vi "字符键盘.vi"(11 "Old String":string) -> (3 "String":string)   [LabVIEW 2016, in "Alarm interface.lvlib" / "短信语音库.lvlib"]
uses:
  <vilib>/Utility/miscctls.llb/LVPointTypeDef.ctl
panel:
  in  "^":bool
  in  "$":bool
  in  "!":bool
  in  "~":bool
  in  "%":bool
  in  "&":bool
  in  "@":bool
  in  "_":bool
  in  "#":bool
  in  "大小写":bool
  in  "Z":bool
  in  "Y":bool
  in  "X":bool
  in  "W":bool
  in  "V":bool
  in  "U":bool
  in  "T":bool
  in  "S":bool
  in  "R":bool
  in  "Q":bool
  in  "P":bool
  in  "O":bool
  in  "N":bool
  in  "M":bool
  in  "L":bool
  in  "K":bool
  in  "J":bool
  in  "I":bool
  in  "H":bool
  in  "G":bool
  in  "F":bool
  in  "E":bool
  in  "D":bool
  in  "C":bool
  in  "B":bool
  in  "A":bool
  in  ",":bool
  in  "Cancel":bool
  in  "OK":bool
  in  "Clear":bool
  in  "BackSpace":bool
  in  "Point":bool
  in  "Zero":bool
  in  "Nine":bool
  in  "Eight":bool
  in  "Seven":bool
  in  "Six":bool
  in  "Five":bool
  in  "Four":bool
  in  "Three":bool
  in  "Two":bool
  in  "One":bool
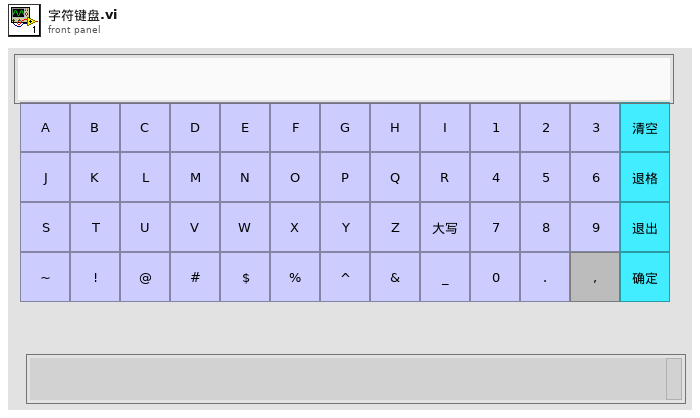
[diagram p1: front panel]
types:
  T1 = typedef "LVPointTypeDef.ctl" = cluster{"Horizontal":i16, "Vertical":i16}
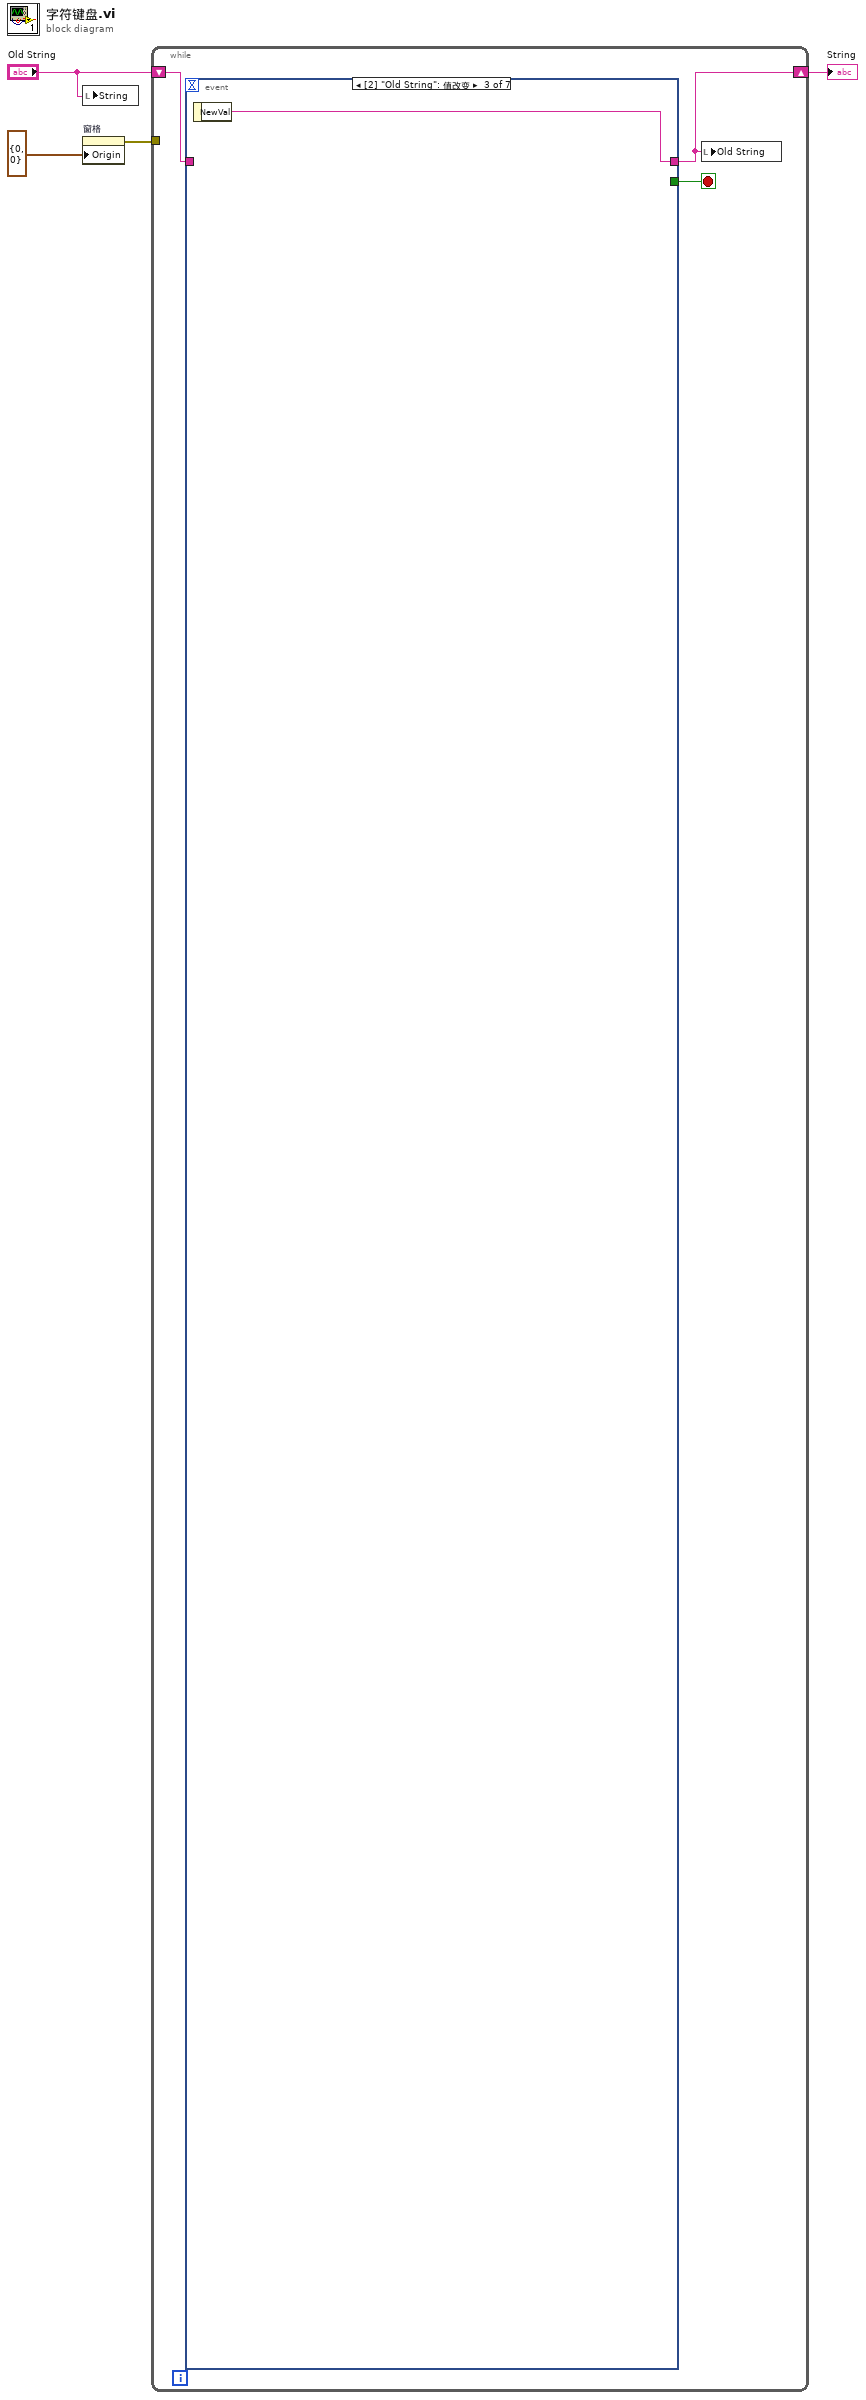
[diagram p0: block diagram]
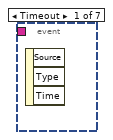
[diagram p2: hidden frame]
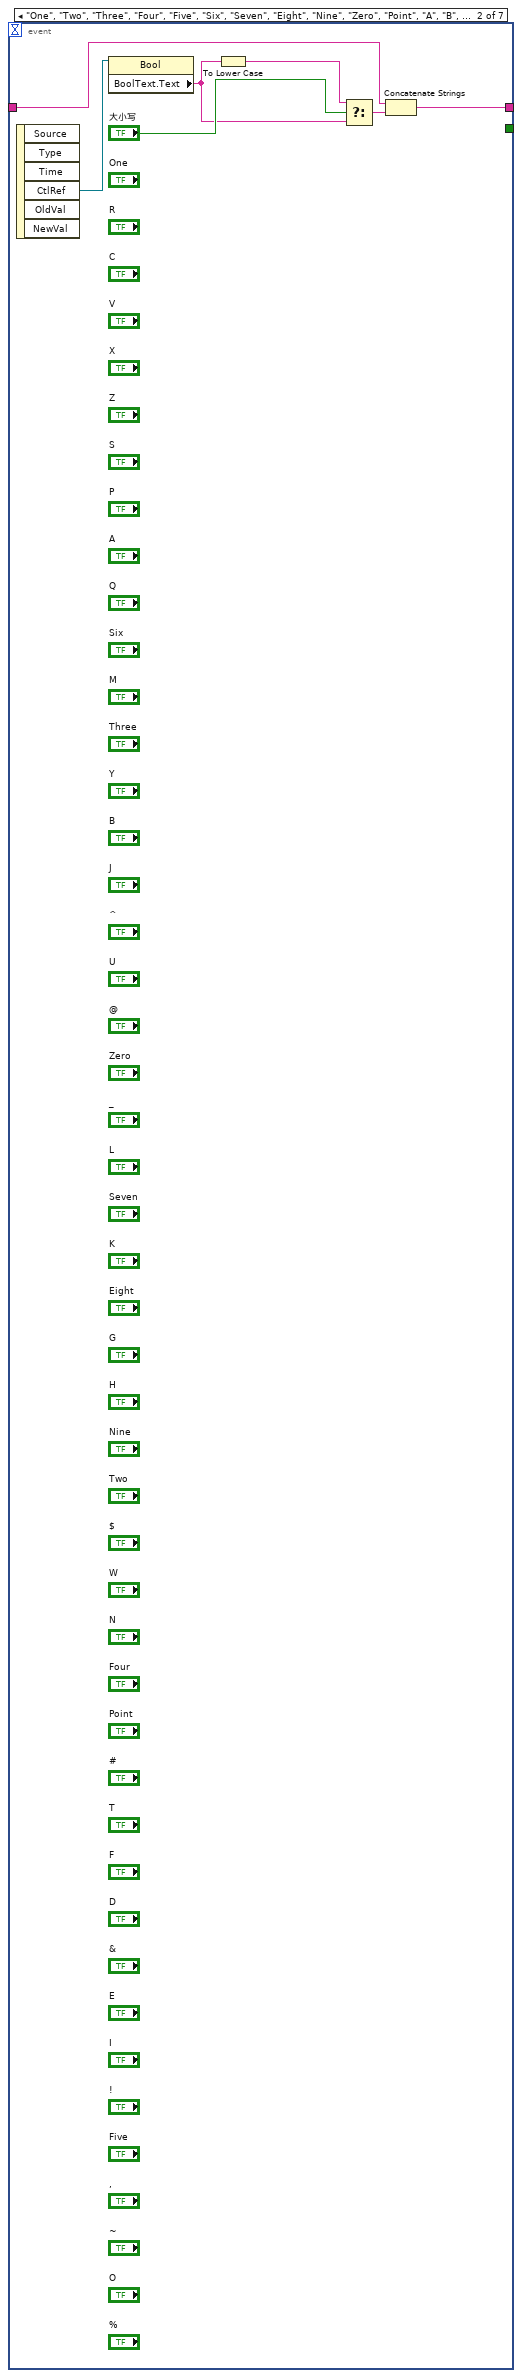
[diagram p3: hidden frame]
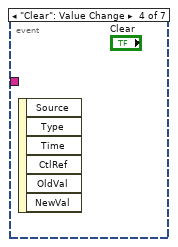
[diagram p4: hidden frame]
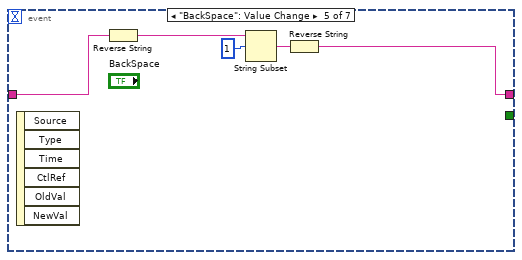
[diagram p5: hidden frame]
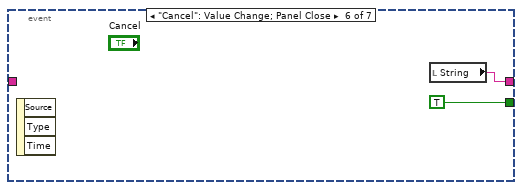
[diagram p6: hidden frame]
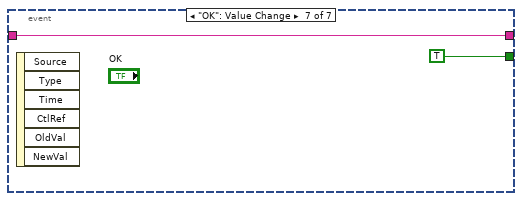
[diagram p7: hidden frame]
diagram:
  n1 = local write "String"("Old String") -> ()
  n2 = property on="窗格" class="Pane"("Origin"=T1 {"Horizontal"=0, "Vertical"=0} ("原点")) -> (error out=w2:errorcluster)  [unwired: 2 in, 1 out]
  n3 = while {
    shift-right: [w5] -> w1
    shift-left: "Old String" -> [w7]
    tunnel: w2 -> [_]
    stop <- w6 stop-if-true
    n4 = event shown="[2] \"Old String\": 值改变" {
      selector: _ -> [_ _ _ _ _ _ _]
      dyn-events: _ -> [_ _ _ _ _ _ _]
      timeout: _ -> [_ _ _ _ _ _ _]
      tunnel: w7 -> [_ w13 _ _ w19 _ w24]
      tunnel: [_ w12 w15 _ w16 w22 w24] -> w5
      tunnel: [_ _ _ _ _ TRUE TRUE] -> w6
      event Timeout {
        n5 = event-data() -> ()  [unwired: 1 in, 3 out]
      }
      event "One", "Two", "Three", "Four", "Five", "Six", "Seven", "Eight", "Nine", "Zero", "Point", "A", "B", "C", "D", "E", "F", "G", "H", "I", "J", "K", "L", "M", "N", "O", "P", "Q", "R", "S", "T", "U", "V", "W", "X", "Y", "Z", "#", "_", "@", "&", "%", "~", "!", "$", "^", ",": Value Change {
        n6 = event-data() -> ("CtlRef"=w14:refnum<vi>)  [unwired: 1 in, 5 out]
        n7 = property class="Bool"(reference=w14) -> ("BoolText.Text"=w8:string)  [unwired: 1 in, 2 out]
        n8 = To Lower Case(string=w8) -> (all lower case string=w9:string)
        n9 = Select(t=w9, s="大小写", f=w8) -> (s? t:f=w10:string)
        n10 = Concatenate Strings(w13, w10) -> (w12:string)
      }
      event "Old String": Value Change {
        n11 = event-data() -> ("NewVal"=w15:string)  [unwired: 1 in]
      }
      event "Clear": Value Change {
        n12 = event-data() -> ()  [unwired: 1 in, 6 out]
      }
      event "BackSpace": Value Change {
        n13 = event-data() -> ()  [unwired: 1 in, 6 out]
        n14 = Reverse String(1:w19) -> (0:w18:string)
        n15 = String Subset(string=w18, offset (0)=1 ("偏移量(0)")) -> (substring=w17:string)  [unwired: 1 in]
        n16 = Reverse String(1:w17) -> (0:w16:string)
      }
      event "Cancel": Value Change; Panel Close {
        n17 = event-data() -> ()  [unwired: 1 in, 3 out]
        n18 = local read "String"() -> (w22:string)
      }
      event "OK": Value Change {
        n19 = event-data() -> ()  [unwired: 1 in, 6 out]
      }
    }
    n20 = local write "Old String"(w5) -> ()
  }
  "String" <- w1
